vi "Test exprParser.vi"() -> ()   [LabVIEW 2015]
uses:
  <vilib>/LAVA/AlmostEqual/AlmostEqual_ULPs_DBL.vi
  <vilib>/LAVA/Robust CSV/Robust CSV.lvlib
  <vilib>/LAVA/AlmostEqual/AlmostEqual.lvlib
  <vilib>/gmath/NI_Gmath.lvlib
panel:
  out "Variables":cluster{string, dbl}[](array[cluster]) {"?" format="%_20e"}
  out "NumTests":i32
  out "Failed cases":cluster{string, dbl, "Result":dbl, dbl}[](array[cluster]) {"?" format="%_20e"; "Result" format="%_20e"; "?" format="%_20e"}
  out "NumFails":i32
  in  "Tolerance (ULPs)":u32=100
  out "Test Cases":T1(array[cluster]) {"?" format="%_20e"; "Result" format="%_20e"}
  in  "file path in":path=path "eqTestCases.csv"
  # "Notes:"
  # "muParser evaluates exponents from right to left\na^2^3 = a^(2^3)\nexcel evaluates exponents left to right\na^2^3 = (a^2)^3"
  # "muParser log is base e\n_e^log(a) = a\nexcel log is base 10\n10^log(a) = a"
  # "Expected"
  # "Actual"
  # "Difference"
  # "Expected Result"
  # "Actual Result"
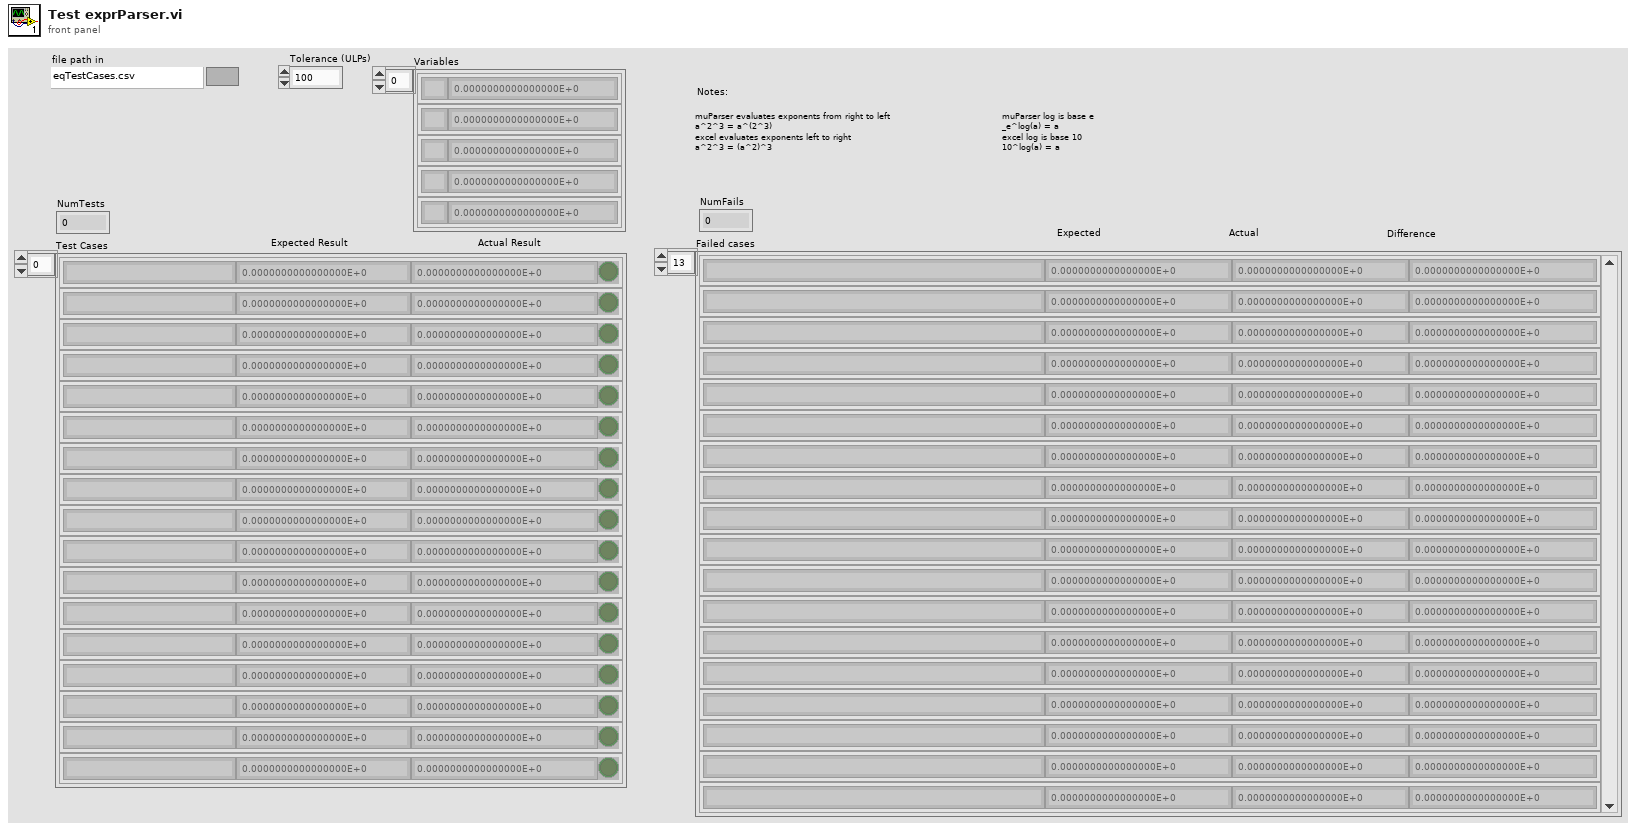
[diagram p1: front panel]
types:
  T1 = cluster{string, dbl, "Result":dbl, "X = Y +/- #ULPs?":bool}[]
  T2 = cluster{string, dbl, "y value":dbl, "X = Y +/- #ULPs?":bool}
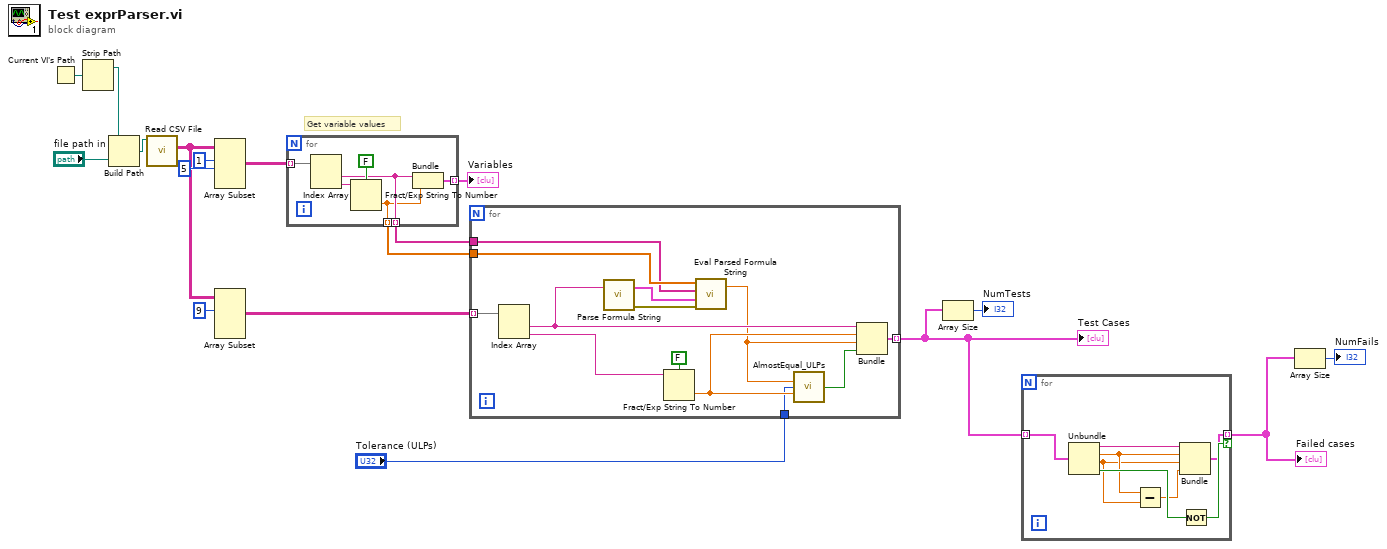
[diagram p0: block diagram]
diagram:
  # "Get variable values"
  n1 = Current VI's Path() -> (path=w4:path)
  n2 = Strip Path(path=w4) -> (stripped path=w2:path)  [unwired: 1 out]
  n3 = Build Path(base path=w2, name or relative path="file path in") -> (appended path=w1:path)
  n4 = call <vilib>:"Read CSV File.vi"("file path in"=w1) -> ("2-D array"=w15:string[][])  [unwired: 8 in, 2 out]
  n5 = Array Subset(array=w15, index (row)=1 ("index"), length (row)=5 ("length")) -> (w16:string[][])  [unwired: 2 in]
  n6 = Array Subset(array=w15, index (row)=9 ("index")) -> (w13:string[][])  [unwired: 3 in]
  n7 = for {
    tunnel: w16 -> [w24] mode=indexing
    tunnel: [w21] -> w5 mode=indexing
    tunnel: [w20] -> w7 mode=indexing
    tunnel: [w19] -> w6 mode=indexing
    n8 = Index Array(array=w24) -> (element #1=w20:string, element #2=w23:string)  [unwired: 2 in]
    n9 = Fract/Exp String To Number(use system decimal point (T)=FALSE, string=w23) -> (number=w19:dbl)  [unwired: 2 in, 1 out]
    n10 = Bundle(w20, w19) -> (w21:cluster{string, dbl})  [unwired: 1 in]
  }
  "Variables" <- w5
  n11 = for {
    tunnel: w13 -> [w37] mode=indexing
    tunnel: [w32] -> w9 mode=indexing
    tunnel: "Tolerance (ULPs)" -> [w31]
    tunnel: w7 -> [w26]
    tunnel: w6 -> [w27]
    n12 = Index Array(array=w37) -> (element #1=w28:string, element #2=w35:string)  [unwired: 2 in]
    n13 = call <vilib>:"Parse Formula String.vi"("formula"=w28) -> ("error out"=w30:errorcluster, "Parsed Formula"=w29:cluster{"Table":i32[][], "Y Values":dbl[]})  [unwired: 1 in]
    n14 = Fract/Exp String To Number(use system decimal point (T)=FALSE, string=w35) -> (number=w34:dbl)  [unwired: 2 in, 1 out]
    n15 = call <vilib>:"Eval Parsed Formula String.vi"("error in (no error)"=w30, "Parsed Formula"=w29, "Variables"=w26, "X Values"=w27) -> ("y value"=w25:dbl)  [unwired: 1 out]
    n16 = call-poly <vilib>:"AlmostEqual_ULPs.vi"("X"=w25, "Tolerance (5 ULPs)"=w31, "Y"=w34) -> ("X = Y +/- #ULPs?"=w33:bool)  [unwired: 12 in]
    n17 = Bundle(w28, w34, "y value"=w25, "X = Y +/- #ULPs?"=w33) -> (w32:T2)  [unwired: 1 in]
  }
  "Test Cases" <- w9
  n18 = Array Size(array=w9) -> (size(s)=→"NumTests":i32)
  n19 = for {
    tunnel: w9 -> [w45] mode=indexing
    tunnel: [w38] -> w11 mode=indexing if=w43
    n20 = Unbundle(w45) -> (w42:string, w41:dbl, "y value"=w40:dbl, "X = Y +/- #ULPs?"=w44:bool)
    n21 = Subtract(x=w41, y=w40) -> (x-y=w39:dbl)
    n22 = Bundle(w42, w41, "y value"=w40, w39) -> (w38:cluster{string, dbl, "y value":dbl, dbl})  [unwired: 1 in]
    n23 = Not(x=w44) -> (.not. x?=w43:bool)
  }
  "Failed cases" <- w11
  n24 = Array Size(array=w11) -> (size(s)=→"NumFails":i32)
